vi "Actor Core.vi"(8 "error in":errorcluster, 11 "MockModel in":refnum<class "TestModelManyTopics.lvclass">) -> (0 "error out":errorcluster, 3 "Actor out":refnum<class "Actor.lvclass">)   [LabVIEW 2017, in "TestModels.lvlib" / "TestModelManyTopics.lvclass"]
doc: "(<B>Filename</B>: Actor Framework.lvlib:Actor.lvclass:Actor Core.vi)\n\nReceives messages to the actor, reacts to them, and initiates any error handling that may shut the actor down.\n\nDescendant classes may override this VI to append parallel tasks for the actor to complete while it handles messages. Overrides use the Call Parent Method node."
uses:
  TestModelManyTopics.lvclass
  C:/Git/mva-framework/Framework/IModel/IModel/IModel.lvclass
  <vilib>/ActorFramework/Actor/Actor.lvclass
  <vilib>/ActorFramework/Actor/Actor.lvclass/Actor.ctl
  <vilib>/ActorFramework/Message Enqueuer/Message Enqueuer.lvclass/Message Enqueuer.ctl
  Source/Framework/IModel/IModel/IModel.lvclass/IModel.ctl
  Source/Framework/IMediator/PublishRequest/PublishRequest.lvclass/PublishRequest.ctl
  Source/Framework/AbstractMessages/PreAddressedMsg/PreAddressedMsg.lvclass/PreAddressedMsg.ctl
  Source/Framework/IMediator/IMediator Messages/Publish Msg/Publish Msg.lvclass/Publish Msg.ctl
  Source/Framework/IMediator/IMediator Messages/Publish Msg/Send Pre-Addressed Publish.vi
  Source/Framework/IObserver/IObserver/Read Unique ID.vi
  Source/Framework/IMediator/PublishRequest/Pack Publish Request.vi
  <vilib>/ActorFramework/Message Enqueuer/Enqueue.vi
  Source/Framework/AbstractMessages/PreAddressedMsg/Read Return Address.vi
  <vilib>/ActorFramework/Actor/Read Self Enqueuer.vi
  <vilib>/ActorFramework/Message Enqueuer/Init from Existing Queue.vi
  Source/Framework/IModel/IModel/IModel.lvclass
  C:/Git/mva-framework/Framework/IObserver/IObserver/IObserver.lvclass
  Source/Framework/IObserver/IObserver/IObserver.lvclass
  C:/Program Files (x86)/National Instruments/LabVIEW 2017/vi.lib/ActorFramework/Actor/Actor.lvclass
  Source/Framework/IMediator/IMediator Messages/Publish Msg/Publish Msg.lvclass
  C:/Git/mva-framework/Framework/AbstractMessages/PreAddressedMsg/PreAddressedMsg.lvclass
  C:/Program Files (x86)/National Instruments/LabVIEW 2017/vi.lib/ActorFramework/Message/Message.lvclass
  <vilib>/ActorFramework/Message Priority Queue/Priority Enqueue.vi
  <vilib>/ActorFramework/Message Enqueuer/Message Enqueuer.lvclass
  Source/Framework/IMediator/PublishRequest/PublishRequest.lvclass
panel:
  out "Publication Cycle":i32
  in  "Stop Publisher":bool
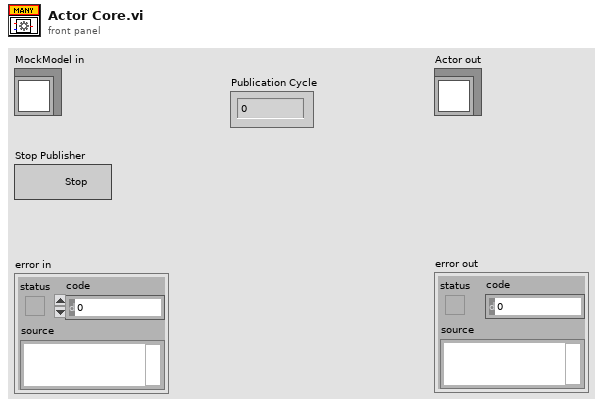
[diagram p1: front panel]
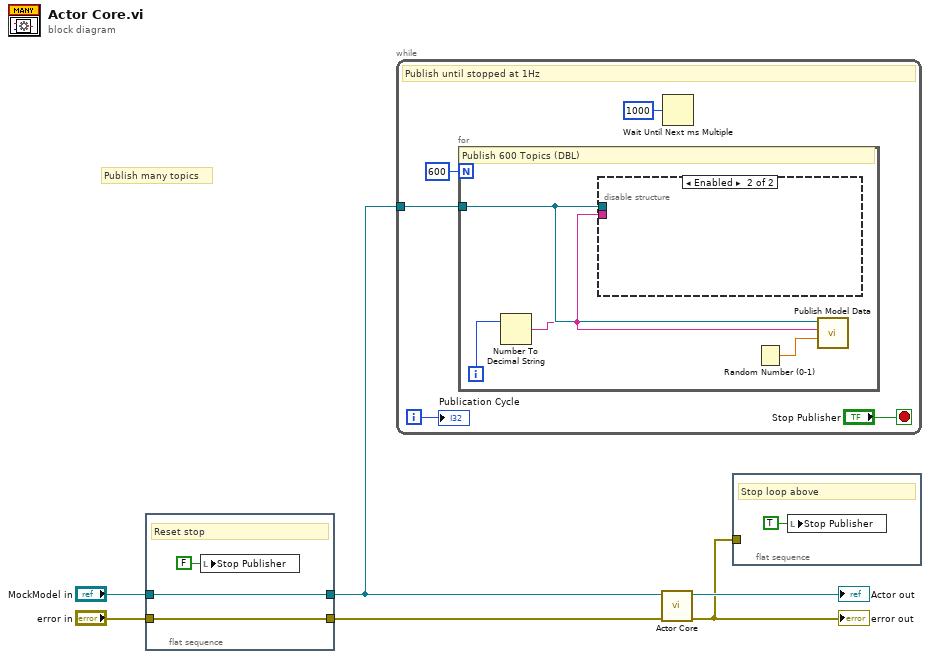
[diagram p0: block diagram]
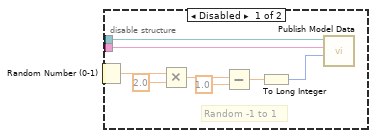
[diagram p2: hidden frame]
diagram:
  # "Publish many topics"
  n1 = flat-sequence {
    tunnel: "MockModel in" -> [w8]
    tunnel: [w8] -> w3
    tunnel: "error in" -> [w7]
    tunnel: [w7] -> w1
    frame #0 {
      # "Reset stop"
      n2 = local write "Stop Publisher"(FALSE ("Stop Publisher")) -> ()
    }
  }
  n3 = while {
    tunnel: w3 -> [w14]
    i -> [w10]
    stop <- "Stop Publisher" stop-if-true
    # "Publish until stopped at 1Hz"
    n4 = for {
      N: 600 -> [_]
      tunnel: w14 -> [w18]
      i -> [w17]
      # "Publish 600 Topics (DBL)"
      n5 = Number To Decimal String(number=w17) -> (decimal integer string=w15:string)  [unwired: 1 in]
      n6 = disable-structure shown="Enabled" {
        disable-tunnel: w18 -> [w26 _]
        disable-tunnel: w15 -> [w25 _]
        frame Disabled {
          # "Random -1 to 1"
          n7 = Random Number (0-1)() -> (number: 0 to 1=w24:dbl)
          n8 = Multiply(x=w24, y=2.0) -> (x*y=w21:dbl)
          n9 = Subtract(x=w21, y=1.0) -> (x-y=w22:dbl)
          n10 = To Long Integer(number=w22) -> (32bit integer=w19:i32)
          n11 = call "Publish Model Data.vi"("Data to Publish"=w19, "Datum Name"=w25, "IModel in"=w26) -> ()  [unwired: 7 in, 2 out]
        }
        frame Enabled {
        }
      }
      n12 = Random Number (0-1)() -> (number: 0 to 1=w16:dbl)
      n13 = call "Publish Model Data.vi"("Data to Publish"=w16, "Datum Name"=w15, "IModel in"=w18) -> ()  [unwired: 7 in, 2 out]
    }
    n14 = Wait Until Next ms Multiple(millisecond multiple=u32 1000) -> ()  [unwired: 1 out]
    "Publication Cycle" <- w10
  }
  n15 = call-parent "Actor Core.vi"("error in"=w1, "Actor in"=w3) -> ("error out"=w5:errorcluster, "Actor out"=→"Actor out":refnum<class "Actor.lvclass">)  [unwired: 8 in]
  "error out" <- w5
  n16 = flat-sequence {
    tunnel: w5 -> [_]
    frame #0 {
      # "Stop loop above"
      n17 = local write "Stop Publisher"(TRUE ("Stop Publisher")) -> ()
    }
  }
